vi "VI Under Test.vi"(10 "N2":dbl=2.0, 11 "N1":dbl=1.0) -> (3 "Result":dbl=3.0)   [LabVIEW 2023]
doc: "This is the VI under test for User-defined Test Advanced.lvtest and User-defined Test Basic.lvtest."
panel:
  # "Overview: This is the VI under test for User-defined Test Advanced.lvtest and User-defined Test Basic.lvtest.\nRequirements: LabVIEW Full Development System, Unit Test Framework Toolkit\nInstructions:\nInstructions:\n1.  Execute the test files for this VI, User-defined Test Advanced.lvtest and User-defined Test Basic.lvtest. In the Project Explorer window, right-click VI under Test.vi to select Unit Tests>>Run from the shortcut menu.\n2.  View the test results in the Unit Test Framework Results window, which shows that the two tests passed during test execution."
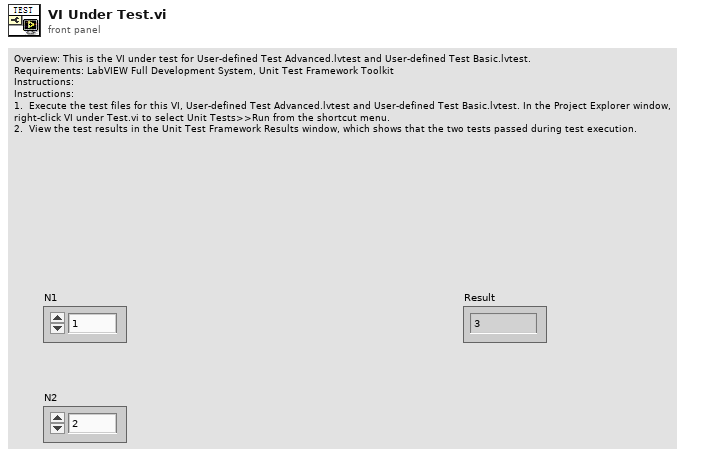
[diagram p1: front panel]
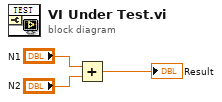
[diagram p0: block diagram]
diagram:
  n1 = Add(x="N1", y="N2") -> (x+y=→"Result":dbl)
